vi "Read BMS request status.vi"(7 "timeout in ms (-1)":i32=-1, 8 "error in":errorcluster, 11 "CAN Session In":T2=refnum) -> (0 "error out":errorcluster, 2 "Stage Request Status":T1, 3 "CAN Session Out":T2)   [LabVIEW 2016]
uses:
  Program Files (x86)/National Instruments/LabVIEW 2016/examples/robotics/EPOS2 CANOpen Driver/Low Level VIs/Typedefs/CAN Refnum.ctl
  Program Files (x86)/National Instruments/LabVIEW 2016/examples/robotics/EPOS2 CANOpen Driver/Low Level VIs/Typedefs/CAN Session Pointer.ctl
  Program Files (x86)/National Instruments/LabVIEW 2016/examples/robotics/EPOS2 CANOpen Driver/Low Level VIs/Typedefs/CAN Communication References.ctl
  Program Files (x86)/National Instruments/LabVIEW 2016/examples/robotics/EPOS2 CANOpen Driver/Low Level VIs/Typedefs/kill process notifier array.ctl
  Program Files (x86)/National Instruments/LabVIEW 2016/examples/robotics/EPOS2 CANOpen Driver/Low Level VIs/Typedefs/Write Queue.ctl
  Program Files (x86)/National Instruments/LabVIEW 2016/examples/robotics/EPOS2 CANOpen Driver/Low Level VIs/Typedefs/FPGA CAN Frame Cluster.ctl
  Stage Request Status.ctl
  Read single CAN.vi
  Data to Stage Request Status.vi
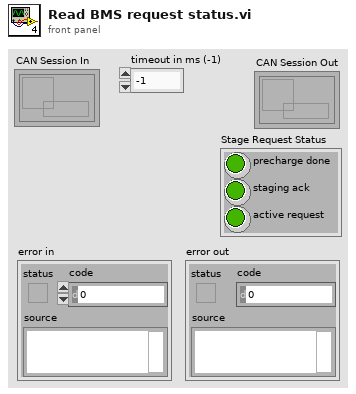
[diagram p1: front panel]
types:
  T1 = typedef "Stage Request Status.ctl" = cluster{"precharge done":bool, "staging ack":bool, "active request":bool}
  T2 = typedef "CAN Refnum.ctl" = refnum<k1>
  T3 = typedef "FPGA CAN Frame Cluster.ctl" = cluster{"Timestamp":u64, "Identifier":u32, "Type":u8, "InfoA":u8, "InfoB":u8, "DataLength":u8, "Data":u8[]}
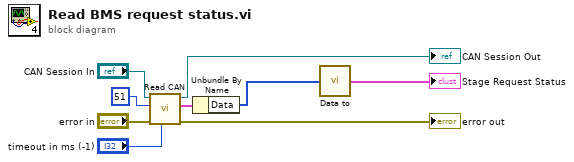
[diagram p0: block diagram]
diagram:
  n1 = call-poly "Read CAN.vi"("timeout in ms (-1)"="timeout in ms (-1)", "error in"="error in", "ID"=51, "CAN Session In"="CAN Session In") -> ("error out"=→"error out":errorcluster, "CAN Frame Out"=w3:T3, "CAN Session Out"=→"CAN Session Out":T2)  [unwired: 5 in]
  n2 = Unbundle By Name(w3) -> ("Data"=w2:u8[])
  n3 = call-poly "Data to.vi"("Data"=w2) -> ("Stage Request Status"=→"Stage Request Status":T1)
